vi "RPM (SubVI).vi"(11 "data in":string) -> (3 "Numeric":dbl)   [LabVIEW 2015]
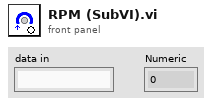
[diagram p1: front panel]
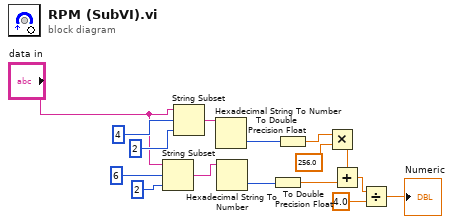
[diagram p0: block diagram]
diagram:
  n1 = String Subset(string="data in", offset (0)=6, length (rest)=2 ("length (rest)")) -> (substring=w15:string)
  n2 = String Subset(string="data in", offset (0)=4, length (rest)=2 ("length (rest)")) -> (substring=w1:string)
  n3 = Hexadecimal String To Number(string=w1) -> (number=w6:u32)  [unwired: 2 in, 1 out]
  n4 = Hexadecimal String To Number(string=w15) -> (number=w5:u32)  [unwired: 2 in, 1 out]
  n5 = To Double Precision Float(number=w5) -> (double precision float=w13:dbl)
  n6 = To Double Precision Float(number=w6) -> (double precision float=w12:dbl)
  n7 = Multiply(x=w12, y=256.0) -> (x*y=w14:dbl)
  n8 = Add(x=w14, y=w13) -> (x+y=w10:dbl)
  n9 = Divide(x=w10, y=4.0) -> (x/y=→"Numeric":dbl)
